vi "Board Transfer.vi"(10 "SystemNumber":string, 11 "connection information":path) -> ()   [LabVIEW 2024]
uses:
  <vilib>/addons/database/Connection.llb/DB Tools Open Connec (Path).vi
  <vilib>/addons/database/Connection.llb/Conn Execute.vi
  <vilib>/addons/database/Recordset.llb/Rec Destroy - Connection.vi
  <vilib>/addons/database/_DB Variant To Data/Database Variant To Data.xnode
  <vilib>/addons/database/NI_Database_API.lvlib
panel:
  out "Lower TimeStart":string
  out "Upper TimeStart":string
  out "NewLowerRackNumber":string
  out "NewSystemNumber":string
  out "NewUpperRackNumber":string
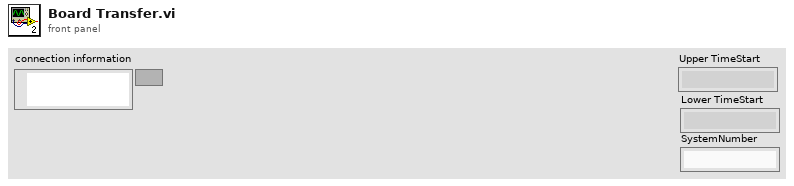
[diagram p1: front panel]
types:
  T1 = typedef "NI_Database_API.lvlib/Conn ObjectReference.ctl" = refnum<k1>
  T2 = typedef "NI_Database_API.lvlib/Rec ObjectReference.ctl" = refnum<k1>
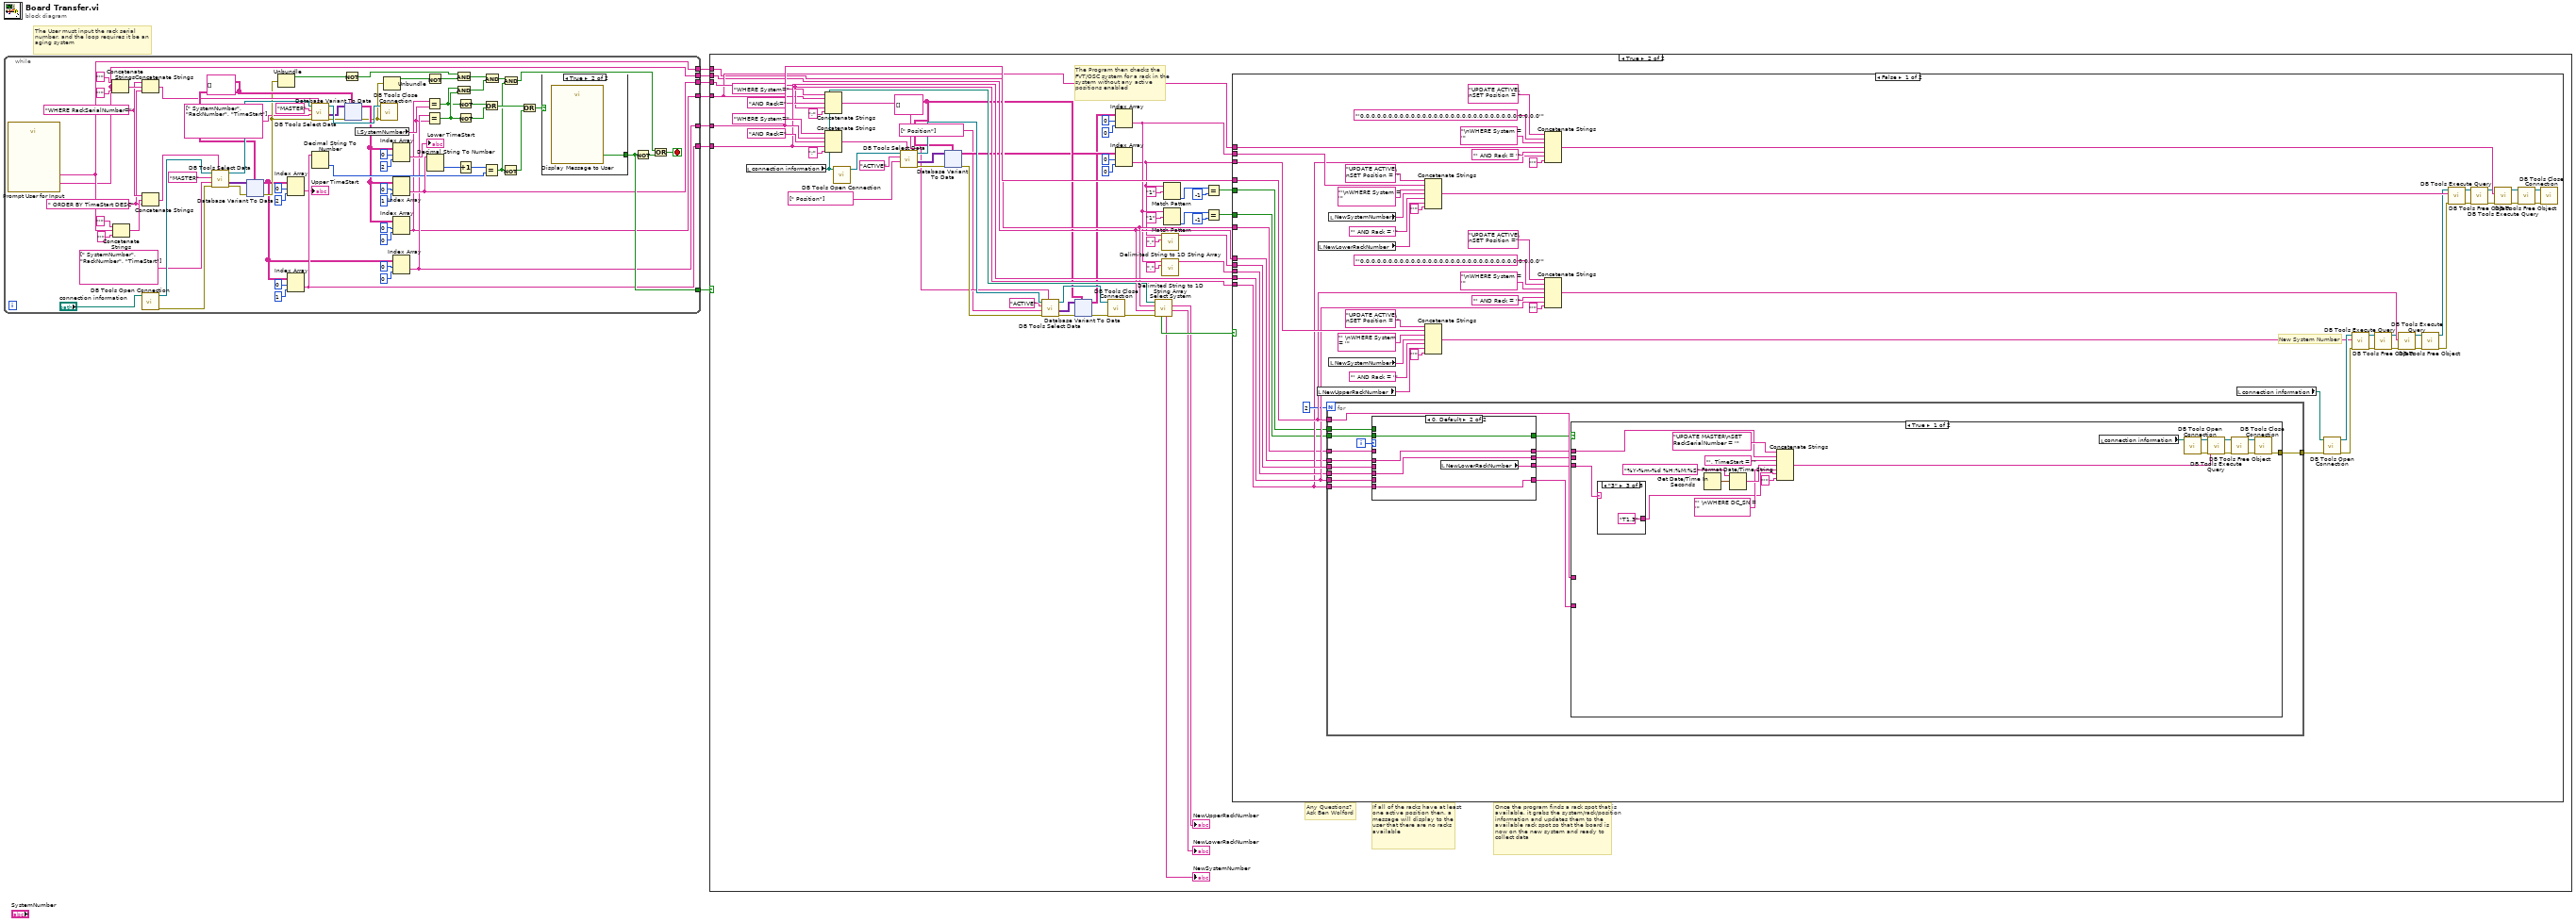
[diagram p0: block diagram]
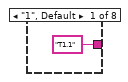
[diagram p3: hidden frame]
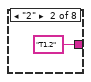
[diagram p4: hidden frame]
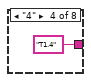
[diagram p5: hidden frame]
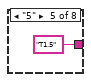
[diagram p6: hidden frame]
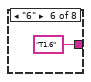
[diagram p7: hidden frame]
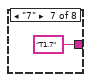
[diagram p8: hidden frame]
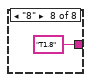
[diagram p9: hidden frame]
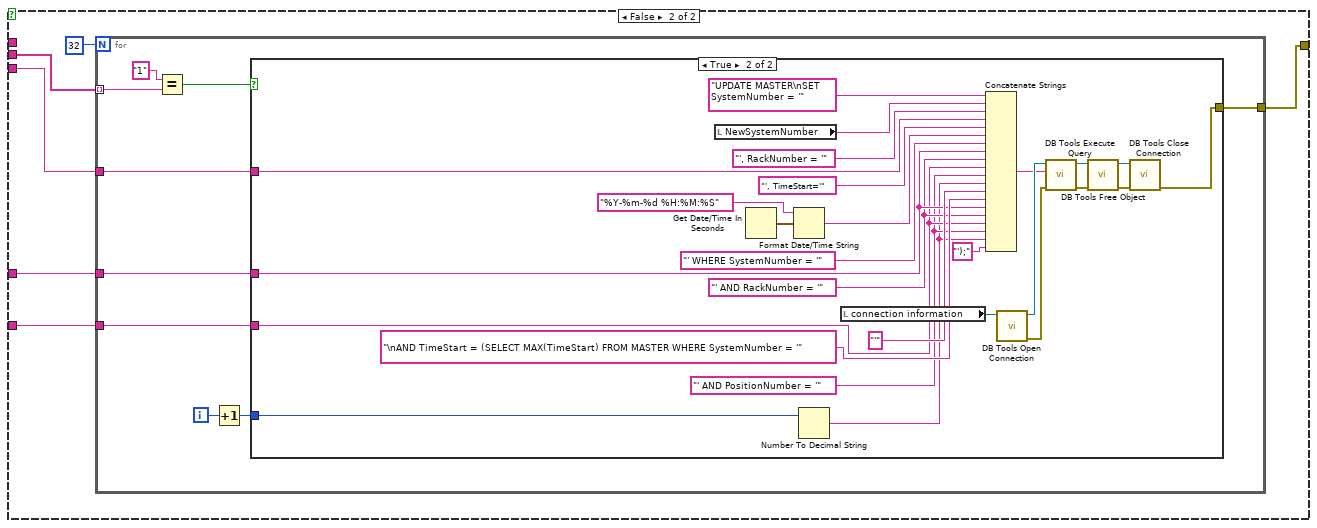
[diagram p10: hidden frame]
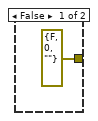
[diagram p11: hidden frame]
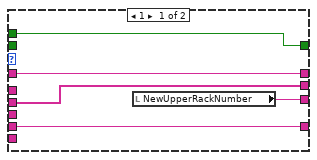
[diagram p12: hidden frame]
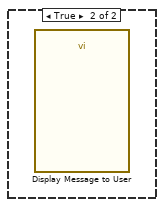
[diagram p13: hidden frame]
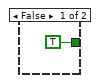
[diagram p14: hidden frame]
diagram:
  # "The User must input the rack serial number, and the loop requires it be an aging system"
  n1 = while {
    tunnel: [w10] -> w7
    tunnel: [w46] -> w6
    tunnel: [w47] -> w3
    tunnel: [w8] -> w2
    tunnel: [w57] -> w5
    tunnel: [w56] -> w4
    tunnel: [w63] -> w1
    stop <- w64 stop-if-true
    w22 = string[][] [] ("string")
    w52 = " ORDER BY TimeStart DESC" ("string")
    w53 = "WHERE RackSerialNumber=" ("SQL Query")
    n2 = call "Prompt User for Input"() -> ("Lower Rack Serial Number"=w56:string, "Upper Rack Serial Number"=w57:string)  [unwired: 16 in, 2 out]
    n3 = Concatenate Strings("'" ("string"), w56, "'" ("string")) -> (w55:string)
    n4 = Concatenate Strings("'" ("string"), w57, "'" ("string")) -> (w54:string)
    n5 = Concatenate Strings(w53, w55, w52) -> (w19:string)
    n6 = Concatenate Strings(w53, w54, w52) -> (w18:string)
    n7 = call-poly <vilib>:"DB Tools Open Connection.vi"("connection information"="connection information") -> ("error out"=w28:errorcluster, "connection reference"=w29:T1)  [unwired: 7 in]
    n8 = call <vilib>:"DB Tools Select Data.vi"("condition"=w18, "error in (no error)"=w28, "columns"=string[] [" SystemNumber", "RackNumber", "TimeStart"], "table"="MASTER" ("ConnectionString In"), "connection reference"=w29) -> ("error out"=w26:errorcluster, "data"=w27:variant[][], "connection reference out"=w30:T1)  [unwired: 1 in]
    n9 = xnode "Database Variant To Data"("database variant"=w27, "error in (no error)"=w26, "type"=w22) -> ("data"=w15:string[][], "error out"=w17:errorcluster)
    n10 = Unbundle(w17) -> ("status"=w78:bool)  [unwired: 2 out]
    n11 = Index Array(array=w15, index (row)=0 ("disabled index (row)"), index (col)=2 ("disabled index (col)")) -> (element=→"Upper TimeStart":string)
    n12 = Index Array(array=w15, index (row)=0, index (col)=1 ("disabled index (col)")) -> (element=w46:string)
    n13 = call <vilib>:"DB Tools Select Data.vi"("condition"=w19, "error in (no error)"=w17, "columns"=string[] [" SystemNumber", "RackNumber", "TimeStart"], "table"="MASTER" ("ConnectionString In"), "connection reference"=w30) -> ("error out"=w23:errorcluster, "data"=w24:variant[][], "connection reference out"=w25:T1)  [unwired: 1 in]
    n14 = Decimal String To Number(string=w46) -> (number=w39:i32)  [unwired: 2 in, 1 out]
    n15 = Not(x=w78) -> (.not. x?=w49:bool)
    n16 = xnode "Database Variant To Data"("database variant"=w24, "error in (no error)"=w23, "type"=w22) -> ("data"=w16:string[][], "error out"=w14:errorcluster)
    n17 = local read "SystemNumber"() -> (w9:string)
    n18 = call <vilib>:"DB Tools Close Connection.vi"("error in (no error)"=w14, "connection reference"=w25) -> ()  [unwired: 5 in, 1 out]
    n19 = Unbundle(w14) -> ("status"=w51:bool)  [unwired: 2 out]
    n20 = Index Array(array=w16, index (row)=0 ("disabled index (row)"), index (col)=2 ("disabled index (col)")) -> (element=→"Lower TimeStart":string)
    n21 = Index Array(array=w16, index (row)=0, index (col)=1 ("disabled index (col)")) -> (element=w47:string)
    n22 = Index Array(array=w16, index (row)=0 ("disabled index (row)"), index (col)=0 ("disabled index (col)")) -> (element=w8:string)
    n23 = Index Array(array=w15, index (row)=0 ("disabled index (row)"), index (col)=0 ("disabled index (col)")) -> (element=w10:string)
    n24 = Equal?(x=w8, y=w9) -> (x = y?=w67:bool)
    n25 = Equal?(x=w10, y=w9) -> (x = y?=w69:bool)
    n26 = Not(x=w51) -> (.not. x?=w48:bool)
    n27 = Decimal String To Number(string=w47) -> (number=w41:i32)  [unwired: 2 in, 1 out]
    n28 = And(x=w49, y=w48) -> (x .and. y?=w50:bool)
    n29 = And(x=w67, y=w69) -> (x .and. y?=w68:bool)
    n30 = Not(x=w67) -> (.not. x?=w66:bool)
    n31 = Not(x=w69) -> (.not. x?=w65:bool)
    n32 = Increment(x=w41) -> (x+1=w40:i32)
    n33 = Or(x=w66, y=w65) -> (x .or. y?=w35:bool)
    n34 = Equal?(x=w40, y=w39) -> (x = y?=w33:bool)
    n35 = And(x=w50, y=w68) -> (x .and. y?=w38:bool)
    n36 = Not(x=w33) -> (.not. x?=w36:bool)
    n37 = And(x=w38, y=w33) -> (x .and. y?=w37:bool)
    n38 = Or(x=w35, y=w36) -> (x .or. y?=w34:bool)
    n39 = case shown="True" w34 {
      tunnel: [TRUE ("OK") w168] -> w63
      frame False {
      }
      frame True {
        n40 = call "Display Message to User"() -> ("OK"=w168:bool)  [unwired: 10 in, 1 out]
      }
    }
    n41 = Not(x=w63) -> (.not. x?=w62:bool)
    n42 = Or(x=w37, y=w62) -> (x .or. y?=w64:bool)
  }
  n43 = case shown="True" w1 {
    tunnel: w7 -> [_ w215]
    tunnel: w6 -> [_ w214]
    tunnel: w5 -> [_ w203]
    tunnel: w4 -> [_ w202]
    tunnel: w3 -> [_ w205]
    tunnel: w2 -> [_ w204]
    frame False {
    }
    frame True {
      w178 = string[][] [] ("string")
      # "Once the program finds a rack spot that is available, it grabs the system/rack/position information and updates them to the available rack spot so that the board is now on the new system and ready to collect data"
      # "If all of the racks have at least one active position then, a message will display to the user that there are no racks available"
      # "Any Questions?\nAsk Ben Wolford"
      # "The Program then checks the FVT/OSC system for a rack in the system without any active positions enabled"
      n44 = local read "connection information"() -> (w186:path)
      n45 = Concatenate Strings("WHERE System=" ("SQL Query"), w204, "AND Rack=", w205, ";" ("string")) -> (w174:string)
      n46 = Concatenate Strings("WHERE System=" ("SQL Query"), w215, "AND Rack=", w214, ";" ("string")) -> (w175:string)
      n47 = call-poly <vilib>:"DB Tools Open Connection.vi"("connection information"=w186) -> ("connection reference"=w188:T1)  [unwired: 7 in, 1 out]
      n48 = call <vilib>:"DB Tools Select Data.vi"("condition"=w175, "columns"=string[] [" Position"], "table"="ACTIVE", "connection reference"=w188) -> ("error out"=w184:errorcluster, "data"=w183:variant[][], "connection reference out"=w187:T1)  [unwired: 2 in]
      n49 = xnode "Database Variant To Data"("database variant"=w183, "error in (no error)"=w184, "type"=w178) -> ("data"=w177:string[][], "error out"=w182:errorcluster)
      n50 = call <vilib>:"DB Tools Select Data.vi"("condition"=w174, "error in (no error)"=w182, "columns"=string[] [" Position"], "table"="ACTIVE", "connection reference"=w187) -> ("error out"=w181:errorcluster, "data"=w179:variant[][], "connection reference out"=w185:T1)  [unwired: 1 in]
      n51 = xnode "Database Variant To Data"("database variant"=w179, "error in (no error)"=w181, "type"=w178) -> ("data"=w176:string[][], "error out"=w180:errorcluster)
      n52 = call <vilib>:"DB Tools Close Connection.vi"("error in (no error)"=w180, "connection reference"=w185) -> ("error out"=w171:errorcluster)  [unwired: 5 in]
      n53 = Index Array(array=w176, index (row)=0, index (col)=0 ("disabled index (col)")) -> (element=w201:string)
      n54 = Index Array(array=w177, index (row)=0, index (col)=0 ("disabled index (col)")) -> (element=w193:string)
      n55 = call "Select System.vi"("Error In"=w171, "LowerRackSerialNumber"=w202, "UpperRackSerialNumber"=w203, "connection information"=w186) -> ("NewLowerRackNumber"=→"NewLowerRackNumber":string, "NewUpperRackNumber"=→"NewUpperRackNumber":string, "NewSystem"=→"NewSystemNumber":string, "Move?"=w206:bool)  [unwired: 3 in, 1 out]
      n56 = call <vilib>:"Delimited String to 1D String Array.vi"("delimiter"=",", "delimited string"=w193) -> ("string array"=w216:string[])  [unwired: 9 in]
      n57 = call <vilib>:"Delimited String to 1D String Array.vi"("delimiter"=",", "delimited string"=w201) -> ("string array"=w207:string[])  [unwired: 9 in]
      n58 = Match Pattern(string=w193, regular expression="1") -> (offset past match=w196:i32)  [unwired: 1 in, 3 out]
      n59 = Match Pattern(string=w201, regular expression="1") -> (offset past match=w199:i32)  [unwired: 1 in, 3 out]
      n60 = Equal?(x=w196, y=-1) -> (x = y?=w192:bool)
      n61 = Equal?(x=w199, y=-1) -> (x = y?=w197:bool)
      n62 = case shown="False" w206 {
        tunnel: w216 -> [w348 _]
        tunnel: w215 -> [w347 _]
        tunnel: w214 -> [w346 _]
        tunnel: w193 -> [w363 _]
        tunnel: w207 -> [w345 _]
        tunnel: w201 -> [w352 _]
        tunnel: w205 -> [w343 _]
        tunnel: w204 -> [w349 _]
        tunnel: w203 -> [w342 _]
        tunnel: w202 -> [w341 _]
        tunnel: w197 -> [w340 _]
        tunnel: w192 -> [w339 _]
        frame False {
          # "New System Number"
          n63 = local read "NewUpperRackNumber"() -> (w364:string)
          n64 = local read "NewLowerRackNumber"() -> (w350:string)
          n65 = for {
            N: 2 -> [_]
            tunnel: w348 -> [w383]
            tunnel: w347 -> [w385]
            tunnel: w346 -> [w381]
            tunnel: w345 -> [w382]
            tunnel: w343 -> [w380]
            tunnel: w342 -> [w373]
            tunnel: w341 -> [w371]
            tunnel: w340 -> [w376]
            tunnel: w339 -> [w374]
            tunnel: [w370] -> w327
            i -> [w384]
            n66 = case shown="0, Default" w384 {
              tunnel: w383 -> [w460 _]
              tunnel: w382 -> [_ w465]
              tunnel: [w460 w465] -> w379
              tunnel: [w459 w464] -> w378
              tunnel: w381 -> [w456 _]
              tunnel: [w456 w461] -> w377
              tunnel: w380 -> [_ w461]
              tunnel: w376 -> [_ w462]
              tunnel: [w457 w462] -> w375
              tunnel: w374 -> [w457 _]
              tunnel: w373 -> [w458 _]
              tunnel: [w458 w463] -> w372
              tunnel: w371 -> [_ w463]
              frame 1 {
                n67 = local read "NewUpperRackNumber"() -> (w459:string)
              }
              frame 0, Default {
                n68 = local read "NewLowerRackNumber"() -> (w464:string)
              }
            }
            n69 = case shown="True" w375 {
              tunnel: w385 -> [_ w418]
              tunnel: w379 -> [_ w416]
              tunnel: w378 -> [w396 w415]
              tunnel: w377 -> [_ w414]
              tunnel: w372 -> [w399 _]
              tunnel: [w390 w413] -> w370
              frame True {
                n70 = case shown="\"3\"" w396 {
                  tunnel: ["T1.1" "T1.2" "T1.3" "T1.4" "T1.5" "T1.6" "T1.7" "T1.8"] -> w397
                  frame "1", Default {
                  }
                  frame "2" {
                  }
                  frame "3" {
                  }
                  frame "4" {
                  }
                  frame "5" {
                  }
                  frame "6" {
                  }
                  frame "7" {
                  }
                  frame "8" {
                  }
                }
                n71 = Get Date/Time In Seconds() -> (seconds since 1Jan1904=w404:timestamp)
                n72 = Format Date/Time String(time format string (%c)="%Y-%m-%d %H:%M:%S", seconds (now)=w404) -> (date/time string=w400:string)  [unwired: 1 in]
                n73 = Concatenate Strings("UPDATE MASTER\nSET RackSerialNumber = '" ("SQL Query"), w399, "', TimeStart = '" ("string"), w400, "' \nWHERE DC_SN = '" ("string"), w397, "'" ("string")) -> (w391:string)
                n74 = local read "connection information"() -> (w392:path)
                n75 = call-poly <vilib>:"DB Tools Open Connection.vi"("connection information"=w392) -> ("error out"=w394:errorcluster, "connection reference"=w393:T1)  [unwired: 7 in]
                n76 = call-poly <vilib>:"DB Tools Execute Query.vi"("error in (no error)"=w394, "SQL query"=w391, "connection reference"=w393) -> ("error out"=w388:errorcluster, "recordset reference"=w389:T2)  [unwired: 5 in]
                n77 = call-poly <vilib>:"DB Tools Free Object.vi"("error in (no error)"=w388, "recordset reference"=w389) -> ("error out"=w386:errorcluster, "connection reference"=w387:T1)  [unwired: 8 in]
                n78 = call <vilib>:"DB Tools Close Connection.vi"("error in (no error)"=w386, "connection reference"=w387) -> ("error out"=w390:errorcluster)  [unwired: 5 in]
              }
              frame False {
                n79 = for {
                  N: 32 -> [_]
                  tunnel: w418 -> [w423]
                  tunnel: w414 -> [w422]
                  tunnel: w416 -> [w421] mode=indexing
                  tunnel: w415 -> [w420]
                  tunnel: [w419] -> w413
                  i -> [w425]
                  n80 = Equal?(x="1", y=w421) -> (x = y?=w426:bool)
                  n81 = Increment(x=w425) -> (x+1=w424:i32)
                  n82 = case shown="True" w426 {
                    tunnel: w424 -> [_ w455]
                    tunnel: w423 -> [_ w443]
                    tunnel: w422 -> [_ w441]
                    tunnel: w420 -> [_ w446]
                    tunnel: [errorcluster {"status"=FALSE, "code"=0, "source"=""} ("error out") w433] -> w419
                    frame False {
                    }
                    frame True {
                      w440 = "' AND PositionNumber = '" ("string")
                      w442 = "' AND RackNumber = '" ("string")
                      n83 = local read "NewSystemNumber"() -> (w451:string)
                      n84 = Get Date/Time In Seconds() -> (seconds since 1Jan1904=w454:timestamp)
                      n85 = Format Date/Time String(time format string (%c)="%Y-%m-%d %H:%M:%S", seconds (now)=w454) -> (date/time string=w449:string)  [unwired: 1 in]
                      n86 = Number To Decimal String(number=w455) -> (decimal integer string=w439:string)  [unwired: 1 in]
                      n87 = local read "connection information"() -> (w435:path)
                      n88 = Concatenate Strings("UPDATE MASTER\nSET SystemNumber = '" ("SQL Query"), w451, "', RackNumber = '" ("string"), w446, "', TimeStart='" ("string"), w449, "' WHERE SystemNumber = '" ("string"), w443, w442, w441, w440, w439, "'" ("string"), "\nAND TimeStart = (SELECT MAX(TimeStart) FROM MASTER WHERE SystemNumber = '" ("string"), w443, w442, w441, w440, w439, "');" ("string")) -> (w434:string)
                      n89 = call-poly <vilib>:"DB Tools Open Connection.vi"("connection information"=w435) -> ("error out"=w437:errorcluster, "connection reference"=w436:T1)  [unwired: 7 in]
                      n90 = call-poly <vilib>:"DB Tools Execute Query.vi"("error in (no error)"=w437, "SQL query"=w434, "connection reference"=w436) -> ("error out"=w431:errorcluster, "recordset reference"=w432:T2)  [unwired: 5 in]
                      n91 = call-poly <vilib>:"DB Tools Free Object.vi"("error in (no error)"=w431, "recordset reference"=w432) -> ("error out"=w429:errorcluster, "connection reference"=w430:T1)  [unwired: 8 in]
                      n92 = call <vilib>:"DB Tools Close Connection.vi"("error in (no error)"=w429, "connection reference"=w430) -> ("error out"=w433:errorcluster)  [unwired: 5 in]
                    }
                  }
                }
              }
            }
          }
          n93 = local read "NewSystemNumber"() -> (w351:string)
          n94 = local read "NewSystemNumber"() -> (w365:string)
          n95 = Concatenate Strings("UPDATE ACTIVE\nSET Position = '" ("SQL Query"), w352, "'\nWHERE System = '" ("string"), w351, "' AND Rack = '" ("string"), w350, "'" ("string")) -> (w329:string)
          n96 = Concatenate Strings("UPDATE ACTIVE\nSET Position = '" ("SQL Query"), w363, "' \nWHERE System = '" ("string"), w365, "' AND Rack = '" ("string"), w364, "'" ("string")) -> (w331:string)
          n97 = Concatenate Strings("UPDATE ACTIVE\nSET Position = " ("SQL Query"), "'0,0,0,0,0,0,0,0,0,0,0,0,0,0,0,0,0,0,0,0,0,0,0,0,0,0,0,0,0,0,0,0'" ("string"), "\nWHERE System = '" ("string"), w349, "' AND Rack = '" ("string"), w343, "'" ("string")) -> (w328:string)
          n98 = Concatenate Strings("UPDATE ACTIVE\nSET Position =" ("SQL Query"), "'0,0,0,0,0,0,0,0,0,0,0,0,0,0,0,0,0,0,0,0,0,0,0,0,0,0,0,0,0,0,0,0'" ("string"), "\nWHERE System = '" ("string"), w347, "' AND Rack = '" ("string"), w346, "'" ("string")) -> (w330:string)
          n99 = local read "connection information"() -> (w332:path)
          n100 = call-poly <vilib>:"DB Tools Open Connection.vi"("error in (no error)"=w327, "connection information"=w332) -> ("error out"=w334:errorcluster, "connection reference"=w333:T1)  [unwired: 6 in]
          n101 = call-poly <vilib>:"DB Tools Execute Query.vi"("error in (no error)"=w334, "SQL query"=w331, "connection reference"=w333) -> ("error out"=w325:errorcluster, "recordset reference"=w326:T2)  [unwired: 5 in]
          n102 = call-poly <vilib>:"DB Tools Free Object.vi"("error in (no error)"=w325, "recordset reference"=w326) -> ("error out"=w323:errorcluster, "connection reference"=w324:T1)  [unwired: 8 in]
          n103 = call-poly <vilib>:"DB Tools Execute Query.vi"("error in (no error)"=w323, "SQL query"=w330, "connection reference"=w324) -> ("error out"=w321:errorcluster, "recordset reference"=w322:T2)  [unwired: 5 in]
          n104 = call-poly <vilib>:"DB Tools Free Object.vi"("error in (no error)"=w321, "recordset reference"=w322) -> ("error out"=w319:errorcluster, "connection reference"=w320:T1)  [unwired: 8 in]
          n105 = call-poly <vilib>:"DB Tools Execute Query.vi"("error in (no error)"=w319, "SQL query"=w329, "connection reference"=w320) -> ("error out"=w317:errorcluster, "recordset reference"=w318:T2)  [unwired: 5 in]
          n106 = call-poly <vilib>:"DB Tools Free Object.vi"("error in (no error)"=w317, "recordset reference"=w318) -> ("error out"=w315:errorcluster, "connection reference"=w316:T1)  [unwired: 8 in]
          n107 = call-poly <vilib>:"DB Tools Execute Query.vi"("error in (no error)"=w315, "SQL query"=w328, "connection reference"=w316) -> ("error out"=w314:errorcluster, "recordset reference"=w313:T2)  [unwired: 5 in]
          n108 = call-poly <vilib>:"DB Tools Free Object.vi"("error in (no error)"=w314, "recordset reference"=w313) -> ("error out"=w311:errorcluster, "connection reference"=w312:T1)  [unwired: 8 in]
          n109 = call <vilib>:"DB Tools Close Connection.vi"("error in (no error)"=w311, "connection reference"=w312) -> ()  [unwired: 5 in, 1 out]
        }
        frame True {
          n110 = call "Display Message to User"() -> ()  [unwired: 10 in, 2 out]
        }
      }
    }
  }
